vi "Builder-Set Project Version.vi"(0 "ProjectItem in":refnum<vi>, 7 "Path":path, 11 "error in (no error)":errorcluster) -> (4 "ProjectItem out":refnum<vi>, 8 "revision":i32, 15 "error out":errorcluster)   [LabVIEW 2020]
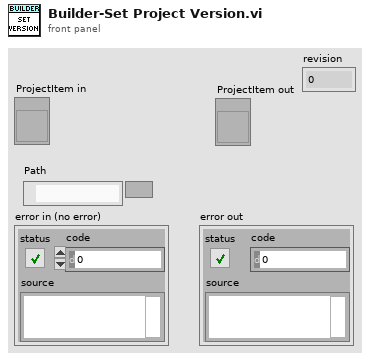
[diagram p1: front panel]
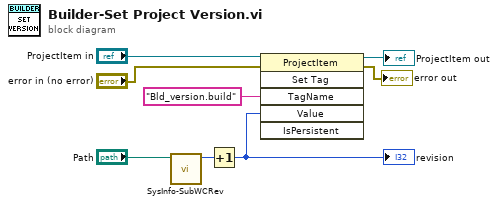
[diagram p0: block diagram]
diagram:
  n1 = call "SysInfo-SubWCRev.vi"("path"="Path") -> ("Revision"=w8:i32)  [unwired: 8 in, 2 out]
  n2 = Increment(x=w8) -> (x+1=w5:i32)
  "revision" <- w5
  n3 = invoke class="ProjectItem" method="Set Tag"(reference="ProjectItem in", error in="error in (no error)", "TagName"="Bld_version.build" ("String"), "Value"=w5) -> (reference out=→"ProjectItem out":refnum<vi>, error out=→"error out":errorcluster)  [unwired: 2 in, 4 out]
